vi "Shutdown.vi"(8 "error in (no error)":errorcluster, 11 "Stage_MadCityLabMicro in":refnum<class "Stage_MadCityLabMicro.lvclass">) -> (0 "error out":errorcluster, 3 "Stage_MadCityLabMicro out":refnum<class "Stage_MadCityLabMicro.lvclass">)   [LabVIEW 2020, in "Stage_MadCityLabMicro.lvlib" / "Stage_MadCityLabMicro.lvclass"]
uses:
  Stage_MadCityLabMicro.lvclass
  Stage_MadCityLabMicro.lvclass/Stage_MadCityLabMicro.ctl
  HAL Layer/Component/Stage/Stage/Stage.lvclass
  Dependency/MicroDrive.dll
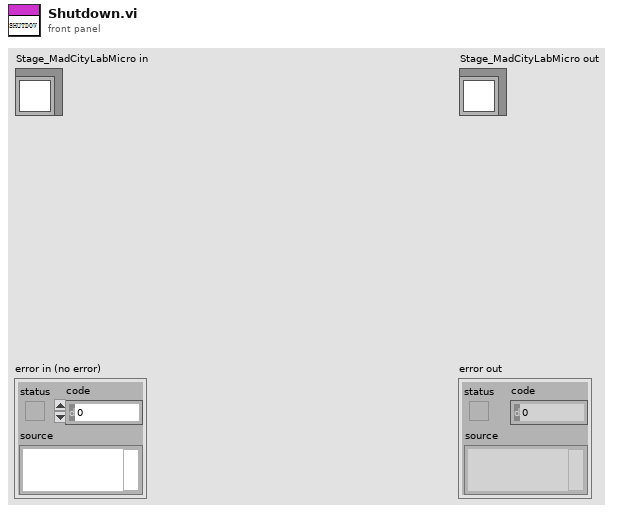
[diagram p1: front panel]
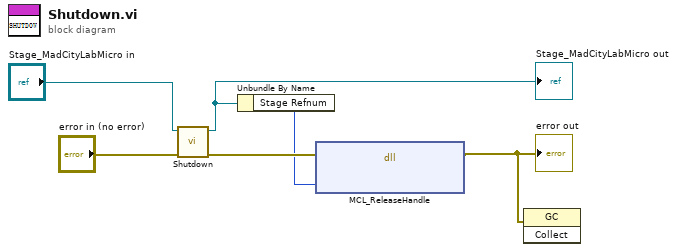
[diagram p0: block diagram]
diagram:
  n1 = call-parent "Shutdown.vi"("error in (no error)"="error in (no error)", "Device in"="Stage_MadCityLabMicro in") -> ("error out"=w4:errorcluster, "Device out"=w3:refnum<class "Stage_MadCityLabMicro.lvclass">)  [unwired: 8 in]
  "Stage_MadCityLabMicro out" <- w3
  n2 = Unbundle By Name(w3) -> ("Stage Refnum"=w2:i32)
  n3 = dll-call lib="D:/Daguan/Development/MMicroscopyAF/Model/Real Hardware/Stage_MadCityLabMicro/Stage_MadCityLabMicro/Dependency/MicroDrive.dll" fn="MCL_ReleaseHandle"(error in=w4, "handle"=w2) -> (error out=w1:errorcluster)  [unwired: 3 in, 2 out]
  "error out" <- w1
  n4 = invoke class="GC" method="Collect"(error in=w1) -> ()  [unwired: 2 in, 3 out]
